vi "Crysound1a_CRY591_Setting.vi"(11 "YTESTER测试数据":T1) -> (3 "YTESTER结论":T2)   [LabVIEW 2017]
uses:
  YtCommon.lvlibp/yt`Step StepBaseInput.ctl
  YtCommon.lvlibp/yt`Step StepResult.ctl
  YtCommon.lvlibp/yt`Step TestData.ctl
  YtCommon.lvlibp/yt`Step System Queue.ctl
  afef007f-dcd1-4f47-8546-b536fdcead1b.vi
  2cdb5281-076e-43db-b3e4-4f534c865916.vi
  3ddae9b3-c194-49f8-abcc-3e64e61855d1.vi
  <vilib>/Instr/_visa.llb/VISA Configure Serial Port (Instr).vi
  YtCommon.lvlibp
panel:
  out "read buffer":string
  in  "YTESTER开放参数":T4={"YTESTER_BaseInput"={"isTest"=FALSE, "isSkip"=FALSE, "StepName"="CRY591通道切换", "OnPass"=enum."Next", "OnFail"=enum."Next", "ReTestNumber"=0.0}, "VISA"="", "切换通道"=enum."A"}
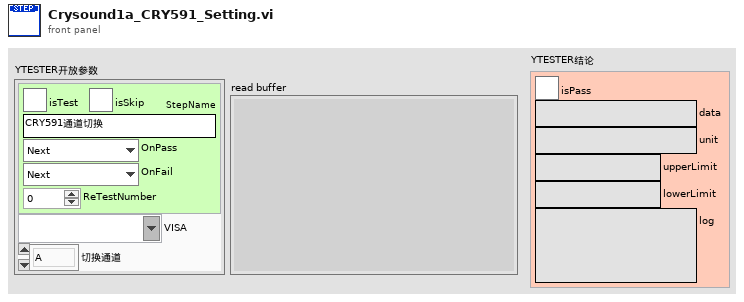
[diagram p1: front panel]
types:
  T1 = typedef "YtCommon.lvlibp/yt`Step TestData.ctl" = cluster{"Socket(From1)":i32, "SN":refnum<notifier>, "StopFlagRef":refnum<notifier>, "YT System Queue":refnum<queue>}
  T2 = typedef "YtCommon.lvlibp/yt`Step StepResult.ctl" = cluster{"isPass":bool, "data":string, "unit":string, "upperLimit":string, "lowerLimit":string, "log":string}
  T3 = typedef "YtCommon.lvlibp/yt`Step StepBaseInput.ctl" = cluster{"isTest":bool, "isSkip":bool, "StepName":string, "OnPass":enum16{"Next", "ToOVER", "Terminate"}, "OnFail":enum16{"Next", "ToOVER", "Terminate"}, "ReTestNumber":dbl}
  T4 = cluster{"YTESTER_BaseInput":T3, "VISA":refnum<visa-resource-name>, "切换通道":enum16{"A", "B"}}
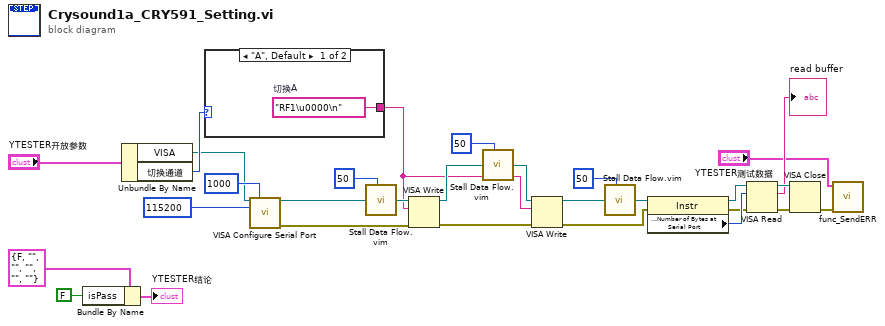
[diagram p0: block diagram]
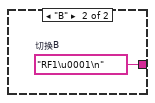
[diagram p2: hidden frame]
diagram:
  n1 = Bundle By Name(cluster=T2 {"isPass"=FALSE, "data"="", "unit"="", "upperLimit"="", "lowerLimit"="", "log"=""} ("Result"), "isPass"=FALSE) -> (→"YTESTER结论":T2)
  n2 = Unbundle By Name("YTESTER开放参数") -> ("VISA"=w1:refnum<visa-resource-name>, "切换通道"=w25:enum16{"A", "B"})
  n3 = case shown="\"A\", Default" w25 {
    tunnel: [w30 w31] -> w5
    frame "A", Default {
      w30 = "RF1\u0000\n"  # 切换A
    }
    frame "B" {
      w31 = "RF1\u0001\n"  # 切换B
    }
  }
  n4 = call-poly "VISA Configure Serial Port"("VISA resource name"=w1, "timeout (10sec)"=u32 1000, "baud rate (9600)"=u32 115200) -> ("VISA resource name out"=w23:refnum<visa-resource-name>, "error out"=w24:errorcluster)  [unwired: 11 in]
  n5 = call "Stall Data Flow.vim"("value in"=w23, "milliseconds to wait"=u32 50) -> ("value out"=w21:refnum<visa-resource-name>)  [unwired: 1 out]
  n6 = VISA Write(VISA resource name=w21, write buffer=w5, error in (no error)=w24) -> (VISA resource name out=w19:refnum<visa-resource-name>, error out=w22:errorcluster)  [unwired: 1 out]
  n7 = call "Stall Data Flow.vim"("value in"=w19, "milliseconds to wait"=u32 50) -> ("value out"=w20:refnum<visa-resource-name>)  [unwired: 1 out]
  n8 = VISA Write(VISA resource name=w20, write buffer=w5, error in (no error)=w22) -> (VISA resource name out=w16:refnum<visa-resource-name>, error out=w9:errorcluster)  [unwired: 1 out]
  n9 = call "Stall Data Flow.vim"("value in"=w16, "milliseconds to wait"=u32 50) -> ("value out"=w15:refnum<visa-resource-name>)  [unwired: 1 out]
  n10 = property class="Instr"(reference=w15, error in=w9) -> (reference out=w14:refnum<visa-resource-name>, error out=w12:errorcluster, "Serial Settings:Number of Bytes at Serial Port"=w13:u32)
  n11 = VISA Read(VISA resource name=w14, byte count=w13, error in (no error)=w12) -> (VISA resource name out=w10:refnum<visa-resource-name>, read buffer=→"read buffer":string, error out=w8:errorcluster)  [unwired: 1 out]
  n12 = VISA Close(VISA resource name=w10, error in (no error)=w8) -> (error out=w3:errorcluster)
  n13 = call "func_SendERR.vi"("ERR (String\\Errclust)"=w3, "YTESTER测试数据 in"="YTESTER测试数据") -> ()  [unwired: 9 in, 1 out]
